vi "GetComputerName.vi"(8 "error in (no error)":errorcluster) -> (0 "error out":errorcluster, 3 "lpbuffer (Computer Name)":string)   [LabVIEW 2018, in "MonSys_Server_Actor.lvlib" / "MonSys_Server_Actor.lvclass"]
doc: "Liest den Computernamen aus"
uses:
  MonSys_Server_Actor.lvclass
  kernel32.dll
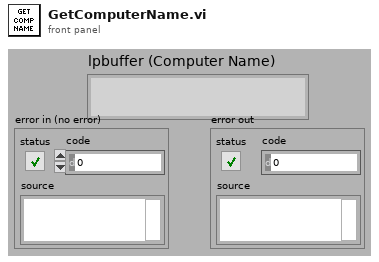
[diagram p1: front panel]
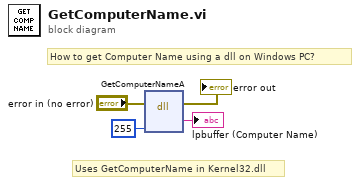
[diagram p0: block diagram]
diagram:
  # "How to get Computer Name using a dll on Windows PC?"
  # "Uses GetComputerName in Kernel32.dll"
  n1 = dll-call lib="kernel32.dll" fn="GetComputerNameA"(error in="error in (no error)", "lpnSize"=u32 255) -> (error out=→"error out":errorcluster, "lpbuffer"=→"lpbuffer (Computer Name)":string)  [unwired: 5 in, 1 out]
